vi "TypeDescriptor_GetDataLengthFromType.vi"(11 "type descriptor":i16[](array[numeric])) -> (2 "Length":u32, 3 "type descriptor dup":i16[](array[numeric]))   [LabVIEW 2013, in "OpenDescriptor.lvlib"]
uses:
  OpenDescriptor.lvlib
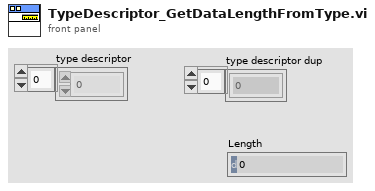
[diagram p1: front panel]
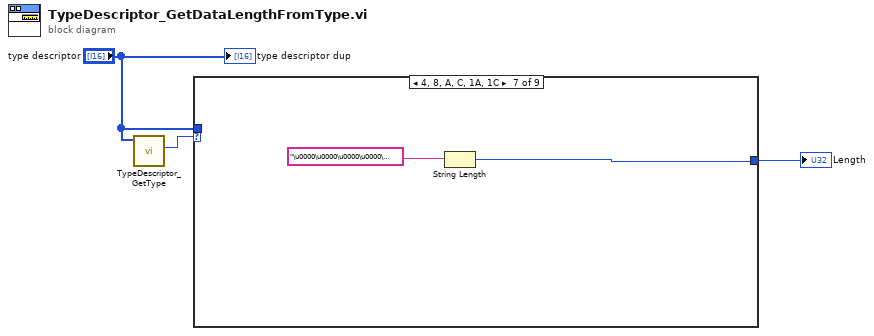
[diagram p0: block diagram]
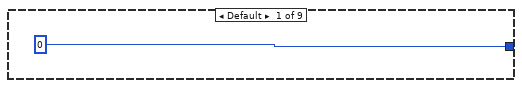
[diagram p2: hidden frame]
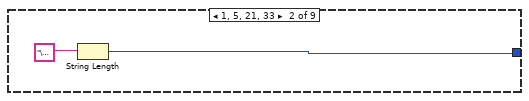
[diagram p3: hidden frame]
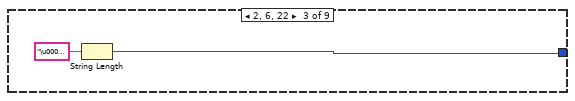
[diagram p4: hidden frame]
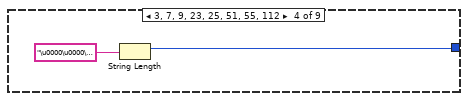
[diagram p5: hidden frame]
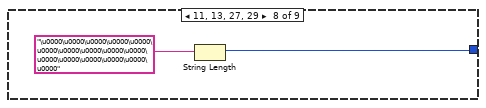
[diagram p8: hidden frame]
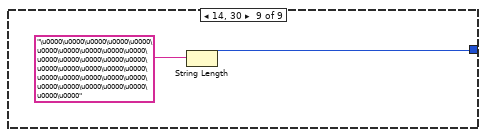
[diagram p9: hidden frame]
diagram:
  n1 = call "TypeDescriptor_GetType.vi"("type descriptor"="type descriptor") -> ("Type"=w3:u8)  [unwired: 9 in, 1 out]
  n2 = case shown="4, 8, A, C, 1A, 1C" w3 {
    tunnel: "type descriptor" -> [_ _ _ _ _ _ _ _ _]
    tunnel: [u32 0 w5 w7 w9 _ _ w11 w13 w16] -> w1
    frame Default {
    }
    frame 1, 5, 21, 33 {
      n3 = String Length(string="\u0000") -> (length=w5:i32)
    }
    frame 2, 6, 22 {
      n4 = String Length(string="\u0000\u0000") -> (length=w7:i32)
    }
    frame 3, 7, 9, 23, 25, 51, 55, 112 {
      n5 = String Length(string="\u0000\u0000\u0000\u0000") -> (length=w9:i32)
    }
    frame 48, 50, 64, 80 {
      # "For clusters (0x50), the length is undefinable from type\nas there might be parts within the cluster that are variable\nlength (strings, arrays, paths, variants, etc.)"
      # "Length is stored in the data string, not the type descriptor"
    }
    frame 83, 84 {
      # "(variant and waveforms)"
      # "Length is stored in the data string, not the type descriptor\nor is variable"
    }
    frame 4, 8, 10, 12, 26, 28 {
      n6 = String Length(string="\u0000\u0000\u0000\u0000\u0000\u0000\u0000\u0000") -> (length=w11:i32)
    }
    frame 11, 13, 27, 29 {
      n7 = String Length(string="\u0000\u0000\u0000\u0000\u0000\u0000\u0000\u0000\u0000\u0000\u0000\u0000\u0000\u0000\u0000\u0000") -> (length=w13:i32)
    }
    frame 14, 30 {
      n8 = String Length(string="\u0000\u0000\u0000\u0000\u0000\u0000\u0000\u0000\u0000\u0000\u0000\u0000\u0000\u0000\u0000\u0000\u0000\u0000\u0000\u0000\u0000\u0000\u0000\u0000\u0000\u0000\u0000\u0000\u0000\u0000\u0000\u0000") -> (length=w16:i32)
    }
  }
  "Length" <- w1
  "type descriptor dup" <- "type descriptor"
